vi "Configure Dwell List.vi"(8 "error in (no error)":errorcluster {"code" format="%.0x"}, 9 "Dwell List":dbl[](array[numeric]) format="%^.3e", 10 "Channel Name (1)":string="1", 11 "VISA resource name":refnum<visa-resource-name>) -> (0 "error out":errorcluster {"code" format="%.0x"}, 3 "VISA resource name out":refnum<visa-resource-name>)   [LabVIEW 2016, in "Agilent N6700 Series.lvlib"]
doc: "Configures the dwell time for each list step.\n\n<b>Note:</b>\nThis VI only applies to models N676xA, N678xA SMU, or models N673xA. N674xA, N675xA, and N677xA with Option 054 (High Speed Test Extensions)."
uses:
  <instrlib>/Agilent N6700 Series/Agilent N6700 Series.lvlib
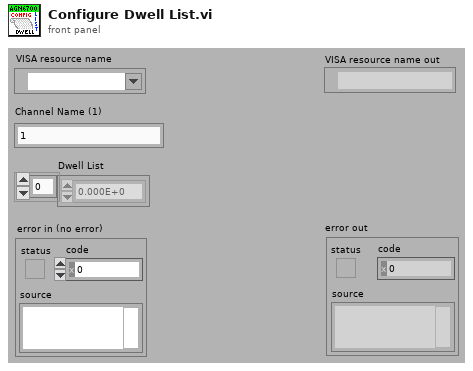
[diagram p1: front panel]
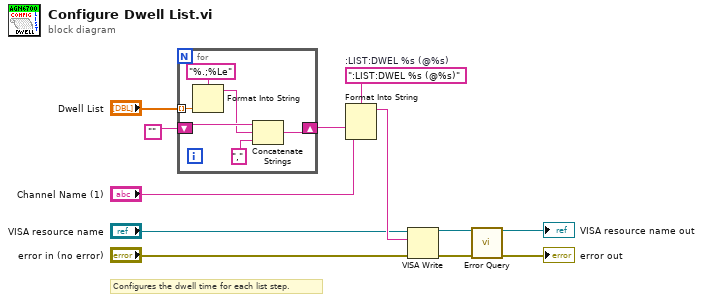
[diagram p0: block diagram]
diagram:
  w12 = ":LIST:DWEL %s (@%s)"  # :LIST:DWEL %s (@%s)
  # "Configures the dwell time for each list step."
  n1 = for {
    tunnel: "Dwell List" -> [w14] mode=indexing
    shift-right: [w18] -> w6
    shift-left: "" -> [w17]
    n2 = Format Into String(format string="%.;%Le", w14) -> (resulting string=w13:string)  [unwired: 2 in, 1 out]
    n3 = Concatenate Strings(w17, w13, ",") -> (w18:string)
  }
  n4 = Format Into String(format string=w12, w6, "Channel Name (1)") -> (resulting string=w11:string)  [unwired: 2 in, 1 out]
  n5 = VISA Write(VISA resource name="VISA resource name", write buffer=w11, error in (no error)="error in (no error)") -> (VISA resource name out=w2:refnum<visa-resource-name>, error out=w1:errorcluster)  [unwired: 1 out]
  n6 = call <instrlib>:"Error Query.vi"("VISA resource name"=w2, "error in (no error)"=w1) -> ("VISA resource name out"=→"VISA resource name out":refnum<visa-resource-name>, "error out"=→"error out":errorcluster)  [unwired: 10 in, 2 out]
